vi "Day 1.2 - Sweep for increasing with average.vi"(11 "input":i32[](array[numeric])) -> (3 "output":i16)   [LabVIEW 2021]
panel:
  out "size(s) 2":i32
  out "size(s)":i32
  out "subarray":i32[](array[numeric])
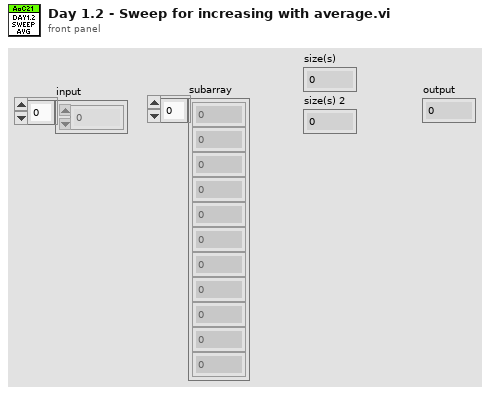
[diagram p1: front panel]
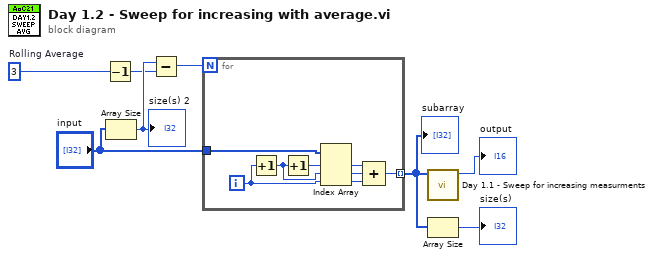
[diagram p0: block diagram]
diagram:
  w7 = 3  # Rolling Average
  n1 = Decrement(x=w7) -> (x-1=w1:i32)
  n2 = Array Size(array="input") -> (size(s)=w8:i32)
  "size(s) 2" <- w8
  n3 = Subtract(x=w8, y=w1) -> (x-y=w6:i32)
  n4 = for {
    N: w6 -> [_]
    tunnel: "input" -> [w16]
    tunnel: [w10] -> w3 mode=indexing
    i -> [w14]
    n5 = Increment(x=w14) -> (x+1=w9:i32)
    n6 = Increment(x=w9) -> (x+1=w15:i32)
    n7 = Index Array(array=w16, index #1=w15, index #2=w9, index #3=w14) -> (element #1=w13:i32, element #2=w11:i32, element #3=w12:i32)
    n8 = Compound Arithmetic op=ADD(w13, w11, w12) -> (w10:i32)
  }
  "subarray" <- w3
  n9 = call "Day 1.1 - Sweep for increasing measurments.vi"("input"=w3) -> ("output"=→"output":i16)  [unwired: 10 in]
  n10 = Array Size(array=w3) -> (size(s)=→"size(s)":i32)
